vi "Calculate Loop Iterations & Period.vi"(11 "Rate":dbl) -> (0 "Wait (ms)":u32, 3 "# Iterations":i32)   [LabVIEW 2015]
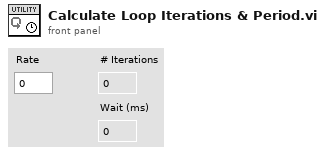
[diagram p1: front panel]
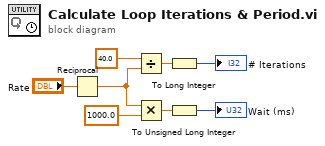
[diagram p0: block diagram]
diagram:
  n1 = Reciprocal(x="Rate") -> (1/x=w7:dbl)
  n2 = Divide(x=40.0, y=w7) -> (x/y=w4:dbl)
  n3 = Multiply(x=w7, y=1000.0) -> (x*y=w3:dbl)
  n4 = To Long Integer(number=w4) -> (32bit integer=→"# Iterations":i32)
  n5 = To Unsigned Long Integer(number=w3) -> (unsigned 32bit integer=→"Wait (ms)":u32)
